vi "NI_XNET_CAN_Bus_Monitor_API InitializeSettings.vi"(6 "contextId":T1, 8 "error in":errorcluster, 9 "timeout (ms)":i32=-1, 10 "Request Data":T4, 11 "gRPC ID":T1) -> (0 "error out":errorcluster, 2 "Response Data":T2, 3 "gRPC ID out":T1)   [LabVIEW 2025, in "xnet_can_bus_monitor_api_client.lvlib"]
uses:
  xnet_can_bus_monitor_api_client.lvlib
  <vilib>/gRPC/LabVIEW gRPC Library/Shared/grpcId.ctl
  RPC Messages/ni_xnet_can_bm_api_InitializeSettingsRequest.ctl
  RPC Messages/ni_xnet_can_bm_api_ConnectSettings.ctl
  RPC Messages/ni_xnet_can_bm_api_CanMode.ctl
  RPC Messages/ni_xnet_can_bm_api_Termination.ctl
  RPC Messages/ni_xnet_can_bm_api_FdIsoMode.ctl
  RPC Messages/ni_xnet_can_bm_api_InitializeSettingsReply.ctl
  RPC Messages/ni_xnet_can_bm_api_ErrorInfo.ctl
  RPC Messages/ni_xnet_can_bm_api_InitializeSettingsReply_Flat.ctl
  RPC Messages/ni_xnet_can_bm_api_ErrorInfo_Flat.ctl
  14035477-4c25-4107-8ed5-d0c4ef420ce5.vi
  RPC Messages/RichToFlatni_xnet_can_bm_api_ConnectSettings.vi
  <vilib>/gRPC/LabVIEW gRPC Library/Shared/TranslateGrpcError.vi
  <vilib>/gRPC/LabVIEW gRPC Library/Shared/Wait On Occurrence.vi
  RPC Messages/FlatToRichni_xnet_can_bm_api_ErrorInfo.vi
  <vilib>/gRPC/LabVIEW gRPC Library/Shared/Is Feature Enabled.vi
  <vilib>/gRPC/LabVIEW gRPC Library/Server API/Server/Get Server DLL Path.vi
  <vilib>/Utility/error.llb/Error Cluster From Error Code.vi
  <vilib>/gRPC/LabVIEW gRPC Library/grpc-lvsupport-release.lvlib
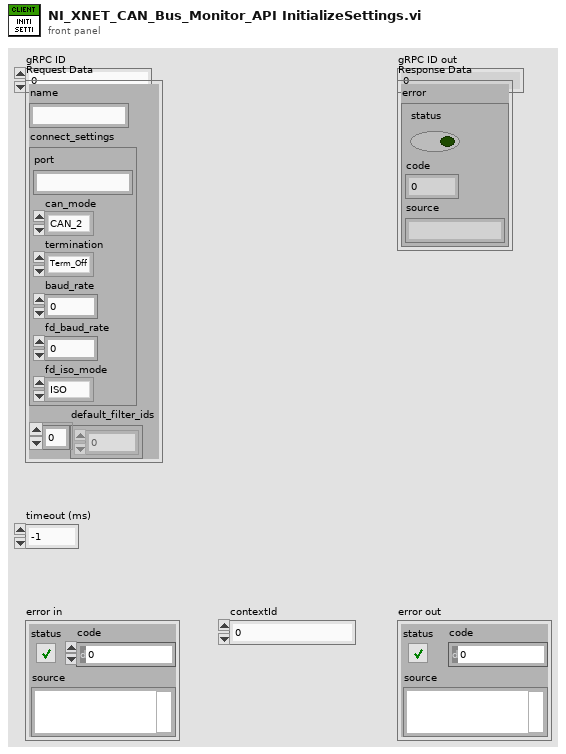
[diagram p1: front panel]
types:
  T1 = typedef "grpc-lvsupport-release.lvlib/grpcId.ctl" = u64
  T2 = typedef "xnet_can_bus_monitor_api_client.lvlib/ni_xnet_can_bm_api_InitializeSettingsReply.ctl" = cluster{"error":T3}
  T3 = typedef "xnet_can_bus_monitor_api_client.lvlib/ni_xnet_can_bm_api_ErrorInfo.ctl" = errorcluster
  T4 = typedef "xnet_can_bus_monitor_api_client.lvlib/ni_xnet_can_bm_api_InitializeSettingsRequest.ctl" = cluster{"name":string, "connect_settings":T5, "default_filter_ids":u32[]}
  T5 = typedef "xnet_can_bus_monitor_api_client.lvlib/ni_xnet_can_bm_api_ConnectSettings.ctl" = cluster{"port":string, "can_mode":T6, "termination":T7, "baud_rate":u64, "fd_baud_rate":u64, "fd_iso_mode":T8}
  T6 = typedef "xnet_can_bus_monitor_api_client.lvlib/ni_xnet_can_bm_api_CanMode.ctl" = enum32{"CAN_2", "CAN_FD", "CAN_FD_BRS"}
  T7 = typedef "xnet_can_bus_monitor_api_client.lvlib/ni_xnet_can_bm_api_Termination.ctl" = enum32{"Term_Off", "Term_On"}
  T8 = typedef "xnet_can_bus_monitor_api_client.lvlib/ni_xnet_can_bm_api_FdIsoMode.ctl" = enum32{"ISO", "Non_ISO", "ISO_Legacy"}
  T9 = typedef "xnet_can_bus_monitor_api_client.lvlib/ni_xnet_can_bm_api_InitializeSettingsReply_Flat.ctl" = cluster{"error":T10}
  T10 = typedef "xnet_can_bus_monitor_api_client.lvlib/ni_xnet_can_bm_api_ErrorInfo_Flat.ctl" = errorcluster
  T11 = typedef "xnet_can_bus_monitor_api_client.lvlib/ni_xnet_can_bm_api_InitializeSettingsRequest_Flat.ctl" = cluster{"name":string, "connect_settings":T12, "default_filter_ids":u32[]}
  T12 = typedef "xnet_can_bus_monitor_api_client.lvlib/ni_xnet_can_bm_api_ConnectSettings_Flat.ctl" = cluster{"port":string, "can_mode":T6, "termination":T7, "baud_rate":u64, "fd_baud_rate":u64, "fd_iso_mode":T8}
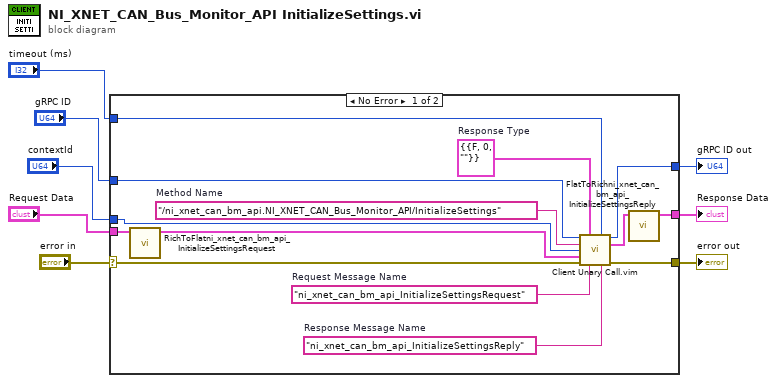
[diagram p0: block diagram]
diagram:
  n1 = case shown="No Error" "error in" {
    selector: "error in" -> [w18 w23]
    tunnel: [w17 w23] -> w7
    tunnel: "gRPC ID" -> [w16 w24]
    tunnel: [w15 w24] -> w5
    tunnel: "Request Data" -> [w12 _]
    tunnel: [w9 _] -> w3
    tunnel: "timeout (ms)" -> [w14 _]
    tunnel: "contextId" -> [w13 _]
    frame No Error {
      w19 = "ni_xnet_can_bm_api_InitializeSettingsReply"  # Response Message Name
      w20 = "ni_xnet_can_bm_api_InitializeSettingsRequest"  # Request Message Name
      w21 = T9 {"error"={"status"=FALSE, "code"=0, "source"=""}}  # Response Type
      w22 = "/ni_xnet_can_bm_api.NI_XNET_CAN_Bus_Monitor_API/InitializeSettings"  # Method Name
      n2 = call "RichToFlatni_xnet_can_bm_api_InitializeSettingsRequest.vi"("InputCluster"=w12) -> ("OutputCluster"=w11:T11)  [unwired: 10 in]
      n3 = call "Client Unary Call.vim"("ClientID in"=w16, "Response Type"=w21, "timeout (ms)"=w14, "Method Name"=w22, "contextId"=w13, "Request Data"=w11, "error in"=w18, "Request Message Name"=w20, "Response Message Name"=w19) -> ("ClientID out"=w15:u64, "Response Data"=w10:T9, "error out"=w17:errorcluster)  [unwired: 4 in]
      n4 = call "FlatToRichni_xnet_can_bm_api_InitializeSettingsReply.vi"("InputCluster"=w10) -> ("OutputCluster"=w9:T2)  [unwired: 10 in]
    }
    frame Error {
    }
  }
  "error out" <- w7
  "gRPC ID out" <- w5
  "Response Data" <- w3
